vi "Magnet Write Message.vi"(7 "Priority Message? (F)":bool, 8 "error in (no error)":errorcluster, 9 "Message Data":variant, 11 "Queue in":refnum<queue>) -> (0 "error out":errorcluster, 3 "Queue out":refnum<queue>)   [LabVIEW 2017, in "Magnet module.lvlib"]
uses:
  Magnet module.lvlib
  ctl/Magnet Orders.ctl
  ctl/MSG to magnet.ctl
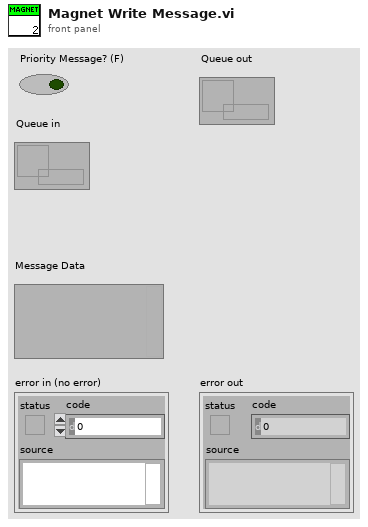
[diagram p1: front panel]
types:
  T1 = typedef "Input message.ctl" = cluster{"Order":T2, "Message Data":variant}
  T2 = typedef "Orders for magnet.ctl" = enum16{"Emergency End", "Initialize", "Update", "Switch mode", "Ramp"}
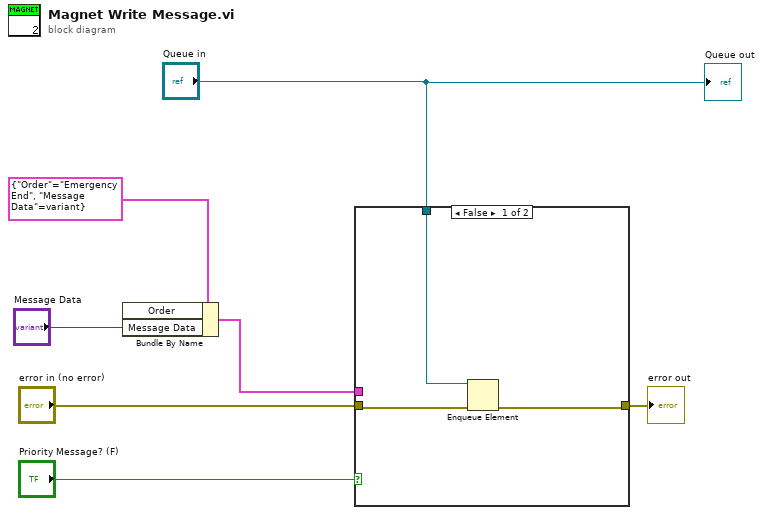
[diagram p0: block diagram]
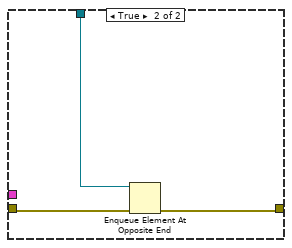
[diagram p2: hidden frame]
diagram:
  n1 = Bundle By Name(cluster=T1 {"Order"=enum."Emergency End", "Message Data"=variant}, "Message Data"="Message Data") -> (w7:T1)  [unwired: 1 in]
  n2 = case shown="False" "Priority Message? (F)" {
    tunnel: "error in (no error)" -> [w9 w13]
    tunnel: [w10 w12] -> w3
    tunnel: "Queue in" -> [w8 w11]
    tunnel: w7 -> [_ _]
    frame False {
      n3 = Enqueue Element(queue=w8, error in (no error)=w9) -> (error out=w10:errorcluster)  [unwired: 2 in, 2 out]
    }
    frame True {
      n4 = Enqueue Element At Opposite End(queue=w11, error in (no error)=w13) -> (error out=w12:errorcluster)  [unwired: 2 in, 2 out]
    }
  }
  "error out" <- w3
  "Queue out" <- "Queue in"
